vi "Config - access supervisory ini file.vi"(5 ".ini Controller":enum16{"Read", "Write"}(ring), 8 "error in":errorcluster, 10 "HLC Controls":T1={"UI Information"={"Header Image"=path "../Data/header.png", "Language"=enum."English", "First Run?"=FALSE, "Setup Camera?"=FALSE, "Device Type"=enum."RCA", "Encoder Type"=enum."Tacho", "Version"=enum."RailMeasurement_CAT", "port"=0, "greyscale"=FALSE, "camera index"=0}, "Test Cluster"={"Operator"="", "Description"="", "Line"="", "Start Position"=450000.0, "Run Length"=31.0, "Sensor A Position"=80000.0, "Rail Side"=FALSE, "Distance Direction"=FALSE, "Path"=path "", "Sensor B Position"=0.0, "Visible Chart Distance"=0.0, "Company"="", "Ref Profile"=""}, "RV-HR Settings Cluster"={"Sensor A Calibration"=0.0, "Integrator Time"=0.0, "Encoder Spacing"=0.0, "Encoder Threshold"=0.0, "Sampling Distance"=0, "Swap Direction?"=FALSE, "Min Walking Speed"=0.0, "Max Walking Speed"=0.0, "Distance Format"=0, "Sensor B Calibration"=0.0, "Tacho Pulses/Rev"=0.0, "Wheel Diameter"=0.0, "Max Short Roughness"=0.0, "Max Long Roughness"=0.0, "Measuring Interval"=0.0, "Measuring Length"=0.0, "Wavelengths"=[], "Device Resolution"=0, "Detect Change in Direction?"=FALSE, "Save Images?"=FALSE, "Image Frequency"=0, "Save Video?"=FALSE, "Image Offset"=0.0, "Start Position at 0m?"=FALSE, "Live Corrug Est.?"=FALSE, "Wavelength Corrug"=0, "Distance Corrug"=0, "Update Corrug"=0}} {"RV-HR Settings Cluster"."Image Frequency" items=["2", "3", "5"]; "RV-HR Settings Cluster"."Device Resolution" items=["0.1 µm", "1 µm", "10 µm"]; "RV-HR Settings Cluster"."Distance Format" items=["kilometres", "miles & chains", "metres", "stations", "miles"]; "RV-HR Settings Cluster"."Sampling Distance" items=["1mm", "2mm"]}, 11 "Config File Ref":T12=refnum) -> (0 "error out":errorcluster, 2 "HLC Controls Out":T1={"UI Information"={"Header Image"=path "../Data/header.png", "Language"=enum."English", "First Run?"=FALSE, "Setup Camera?"=FALSE, "Device Type"=enum."RCA", "Encoder Type"=enum."Tacho", "Version"=enum."RailMeasurement_CAT", "port"=0, "greyscale"=FALSE, "camera index"=0}, "Test Cluster"={"Operator"="", "Description"="", "Line"="", "Start Position"=450000.0, "Run Length"=31.0, "Sensor A Position"=80000.0, "Rail Side"=FALSE, "Distance Direction"=FALSE, "Path"=path "", "Sensor B Position"=0.0, "Visible Chart Distance"=0.0, "Company"="", "Ref Profile"=""}, "RV-HR Settings Cluster"={"Sensor A Calibration"=0.0, "Integrator Time"=0.0, "Encoder Spacing"=0.0, "Encoder Threshold"=0.0, "Sampling Distance"=0, "Swap Direction?"=FALSE, "Min Walking Speed"=0.0, "Max Walking Speed"=0.0, "Distance Format"=0, "Sensor B Calibration"=0.0, "Tacho Pulses/Rev"=0.0, "Wheel Diameter"=0.0, "Max Short Roughness"=0.0, "Max Long Roughness"=0.0, "Measuring Interval"=0.0, "Measuring Length"=0.0, "Wavelengths"=[], "Device Resolution"=0, "Detect Change in Direction?"=FALSE, "Save Images?"=FALSE, "Image Frequency"=0, "Save Video?"=FALSE, "Image Offset"=0.0, "Start Position at 0m?"=FALSE, "Live Corrug Est.?"=FALSE, "Wavelength Corrug"=0, "Distance Corrug"=0, "Update Corrug"=0}} {"RV-HR Settings Cluster"."Image Frequency" items=["2", "3", "5"]; "RV-HR Settings Cluster"."Device Resolution" items=["0.1 µm", "1 µm", "10 µm"]; "RV-HR Settings Cluster"."Distance Format" items=["kilometres", "miles & chains", "metres", "stations", "miles"]; "RV-HR Settings Cluster"."Sampling Distance" items=["1mm", "2mm"]}, 3 "refnum out":T12)   [LabVIEW 2023]
doc: "This subVI reads initial config data from a .ini file to define the default UI.\n\nAuthor: D Keeling\nDate: 20/05/2012\nVersion: 1.0"
uses:
  <vilib>/Utility/config.llb/Config Data RefNum.ctl
  <vilib>/Utility/config.llb/NI_LVConfig.lvlib
  Controls/Supervisory Config Cluster.ctl
  Controls/UI Init Config Info.ctl
  Controls/Test Cluster.ctl
  Controls/Distance Units.ctl
  Controls/Settings Cluster.ctl
  Controls/Sampling DIstance.ctl
  Controls/Language.ctl
  Controls/Device_Type.ctl
  Controls/EncoderType.ctl
  Controls/Device_Resolution.ctl
  Controls/Software Version.ctl
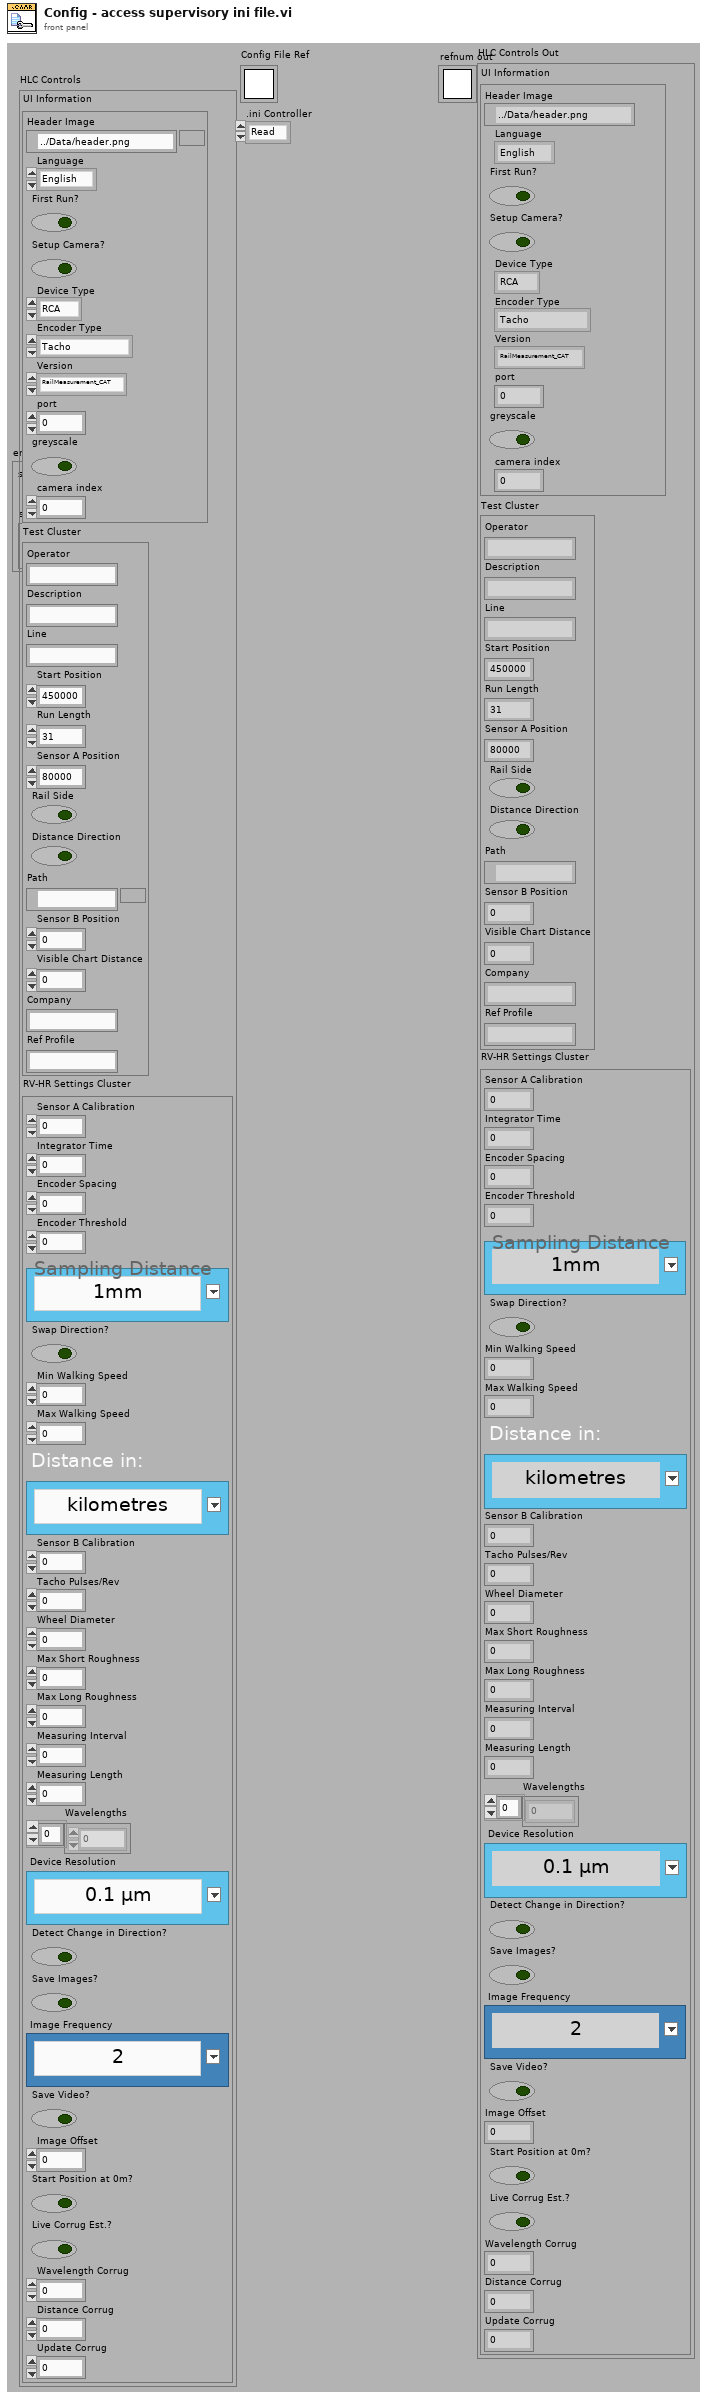
[diagram p1: front panel]
types:
  T1 = typedef "Supervisory Config Cluster.ctl" = cluster{"UI Information":T2, "Test Cluster":T7, "RV-HR Settings Cluster":T8}
  T2 = typedef "UI Init Config Info.ctl" = cluster{"Header Image":path, "Language":T3, "First Run?":bool, "Setup Camera?":bool, "Device Type":T4, "Encoder Type":T5, "Version":T6, "port":i32, "greyscale":bool, "camera index":i32}
  T3 = typedef "Language.ctl" = enum16{"English", "Chinese", "German"}
  T4 = typedef "Device_Type.ctl" = enum16{"CAT", "Bi-CAT", "YRCA", "RCA", "RV-HR", "TV-HR"}
  T5 = typedef "EncoderType.ctl" = enum16{"Tacho", "Quadrature"}
  T6 = typedef "Software Version.ctl" = enum16{"RailMeasurement_CAT", "RailMeasurement_Master", "RailMeasurement_RCA", "RailMeasurement_CAT-V", "RailMeasurement_RCA-V", "RailMeasurement_RV-HR"}
  T7 = typedef "Test Cluster.ctl" = cluster{"Operator":string, "Description":string, "Line":string, "Start Position":dbl, "Run Length":dbl, "Sensor A Position":dbl, "Rail Side":bool, "Distance Direction":bool, "Path":path, "Sensor B Position":dbl, "Visible Chart Distance":dbl, "Company":string, "Ref Profile":string}
  T8 = typedef "Settings Cluster.ctl" = cluster{"Sensor A Calibration":dbl, "Integrator Time":dbl, "Encoder Spacing":dbl, "Encoder Threshold":dbl, "Sampling Distance":T9, "Swap Direction?":bool, "Min Walking Speed":dbl, "Max Walking Speed":dbl, "Distance Format":T10, "Sensor B Calibration":dbl, "Tacho Pulses/Rev":dbl, "Wheel Diameter":dbl, "Max Short Roughness":dbl, "Max Long Roughness":dbl, "Measuring Interval":dbl, "Measuring Length":dbl, "Wavelengths":dbl[], "Device Resolution":T11, "Detect Change in Direction?":bool, "Save Images?":bool, "Image Frequency":T9, "Save Video?":bool, "Image Offset":dbl, "Start Position at 0m?":bool, "Live Corrug Est.?":bool, "Wavelength Corrug":u8, "Distance Corrug":u8, "Update Corrug":u8}
  T9 = typedef "Sampling DIstance.ctl" = u16
  T10 = typedef "Distance Units.ctl" = u16
  T11 = typedef "Device_Resolution.ctl" = u16
  T12 = typedef "NI_LVConfig.lvlib/Config Data RefNum.ctl" = refnum<k1>
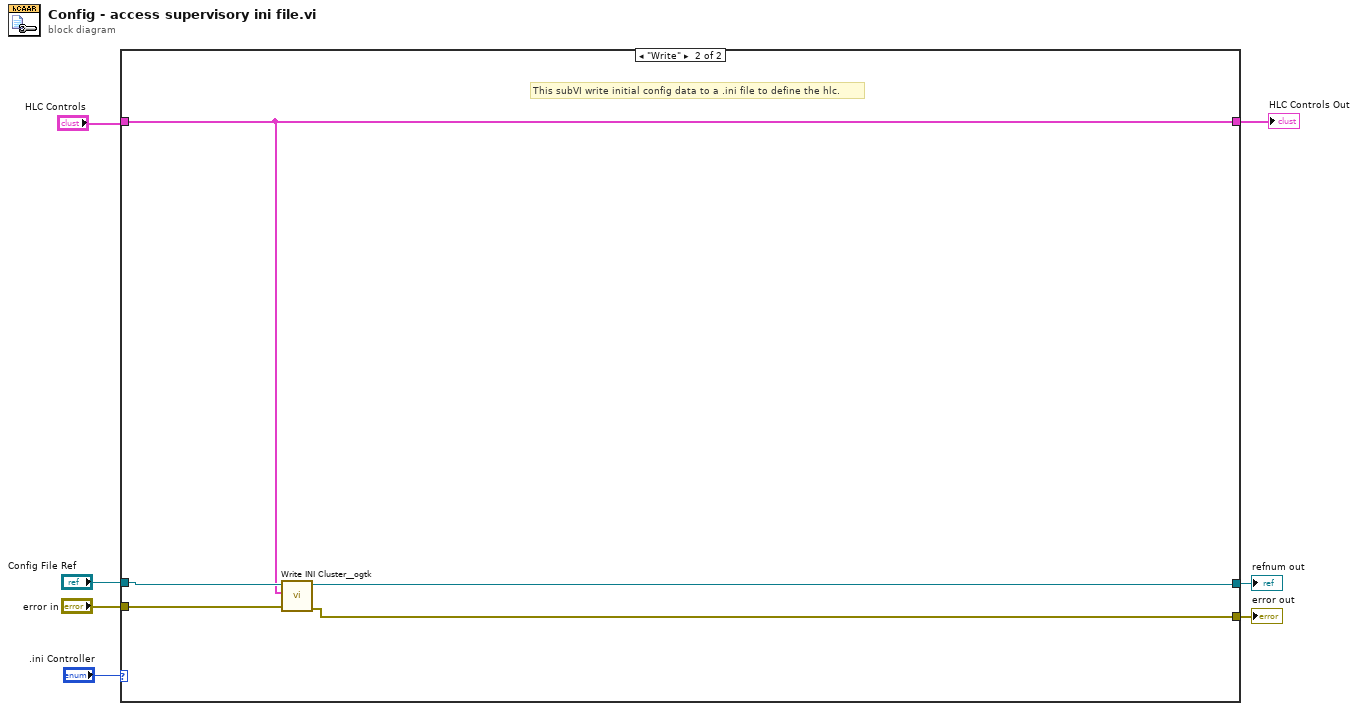
[diagram p0: block diagram]
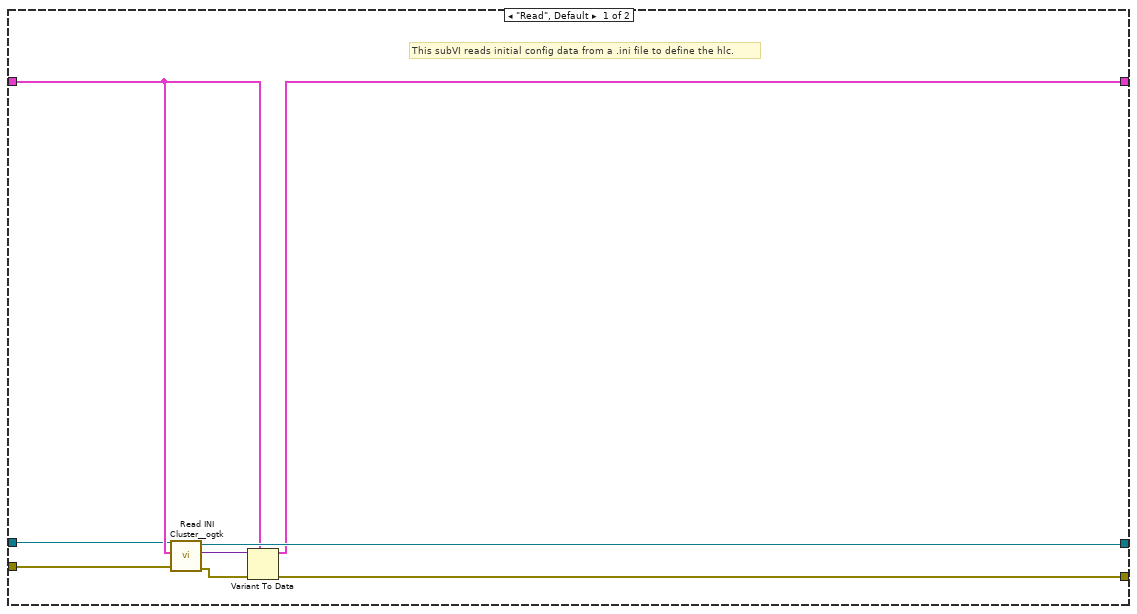
[diagram p2: hidden frame]
diagram:
  n1 = case shown="\"Write\"" ".ini Controller" {
    tunnel: [w14 w20] -> w6
    tunnel: "Config File Ref" -> [w8 w17]
    tunnel: [w15 w19] -> w5
    tunnel: "HLC Controls" -> [w11 w16]
    tunnel: [w10 w16] -> w4
    tunnel: "error in" -> [w9 w18]
    frame "Read", Default {
      # "This subVI reads initial config data from a .ini file to define the hlc."
      n2 = call "Read INI Cluster__ogtk.vi"("error in (no error)"=w9, "INI Fomatted Cluster Type"=w11, "refnum"=w8) -> ("error out"=w12:errorcluster, "INI Fomatted Cluster"=w13:variant, "dup refnum"=w15:T12)  [unwired: 4 in, 2 out]
      n3 = Variant To Data(error in=w12, type=w11, Variant=w13) -> (data=w10:T1, error out=w14:errorcluster)
    }
    frame "Write" {
      # "This subVI write initial config data to a .ini file to define the hlc."
      n4 = call "Write INI Cluster__ogtk.vi"("error in (no error)"=w18, "INI Fomatted Cluster"=w16, "refnum"=w17) -> ("error out"=w20:errorcluster, "dup refnum"=w19:T12)  [unwired: 7 in]
    }
  }
  "error out" <- w6
  "refnum out" <- w5
  "HLC Controls Out" <- w4
